vi "Update Check-in Status.vi"(0 "Guest Manager UI in":refnum<class "Guest Manager UI.lvclass">, 5 "IsSuccess":bool, 7 "Reason If Failure":string, 11 "error in (no error)":errorcluster) -> (4 "Guest Manager UI out":refnum<class "Guest Manager UI.lvclass">, 15 "error out":errorcluster)   [LabVIEW 2023, in "Guest Manager UI.lvlib" / "Guest Manager UI.lvclass"]
uses:
  Guest Manager UI.lvclass
  Guest Manager UI.lvclass/Guest Manager UI.ctl
  <vilib>/ActorFramework/Stop Msg/Stop Msg.lvclass
  <vilib>/ActorFramework/Actor/Actor.lvclass
  C:/Users/bhaghyaraj/Trainings/NI Actor Framework/SDLC/UI Base/UI Base/UI Base.lvclass
  C:/Program Files/National Instruments/LabVIEW 2023/vi.lib/ActorFramework/Actor/Actor.lvclass
  C:/Users/bhaghyaraj/Trainings/NI Actor Framework/SDLC/Guest Manager UI/Guest Manager UI/Guest Manager UI.lvclass
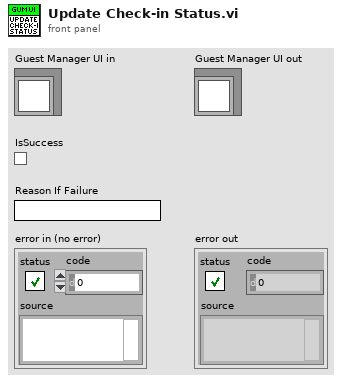
[diagram p1: front panel]
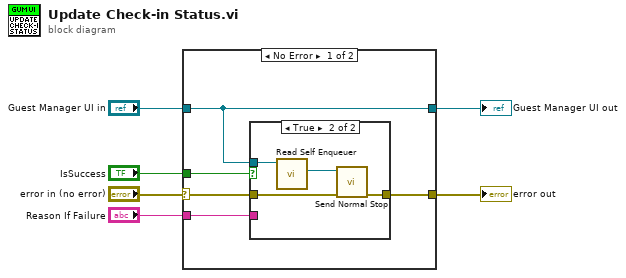
[diagram p0: block diagram]
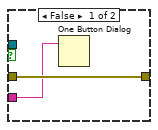
[diagram p2: hidden frame]
diagram:
  n1 = case shown="No Error" "error in (no error)" {
    selector: "error in (no error)" -> [w11 w19]
    tunnel: [w10 w19] -> w5
    tunnel: [w9 w18] -> w3
    tunnel: "Guest Manager UI in" -> [w9 w18]
    tunnel: "IsSuccess" -> [w8 _]
    tunnel: "Reason If Failure" -> [w7 _]
    frame No Error {
      n2 = case shown="True" w8 {
        tunnel: w11 -> [w13 w17]
        tunnel: [w13 w16] -> w10
        tunnel: w9 -> [_ w15]
        tunnel: w7 -> [w12 _]
        frame False {
          n3 = One Button Dialog(message=w12) -> ()  [unwired: 1 in, 1 out]
        }
        frame True {
          n4 = call <vilib>:"Read Self Enqueuer.vi"("Actor"=w15) -> ("Self Enqueuer"=w14:refnum<class "Message Enqueuer.lvclass">)  [unwired: 10 in]
          n5 = call <vilib>:"Send Normal Stop.vi"("error in (no error)"=w17, "Message Enqueuer"=w14) -> ("error out"=w16:errorcluster)  [unwired: 9 in]
        }
      }
    }
    frame Error {
    }
  }
  "error out" <- w5
  "Guest Manager UI out" <- w3
